vi "SigmaSolution.vi"(1 "rou":dbl) -> (0 "sigma":dbl)   [LabVIEW 2014]
uses:
  <vilib>/Analysis/polynomials.llb/Scalar Polynomial Evaluation (DBL).vi
  <vilib>/Analysis/NI_AALPro.lvlib
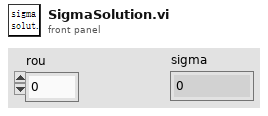
[diagram p1: front panel]
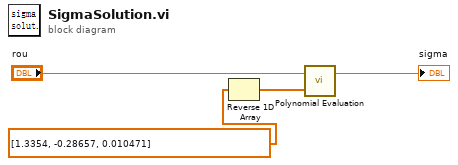
[diagram p0: block diagram]
diagram:
  n1 = Reverse 1D Array(array=dbl[] [1.3354, -0.28657, 0.010471]) -> (reversed array=w1:dbl[])
  n2 = call-poly <vilib>:"Polynomial Evaluation.vi"("P(x)"=w1, "a"="rou") -> ("P(a)"=→"sigma":dbl)  [unwired: 1 out]
